vi "Test_Benchmarking_ManyLogEventCall_AvgCallTimeSub50uS.vi"(8 "error in (no error)":errorcluster, 11 "Benchmarking in":refnum<class "Benchmarking.lvclass">) -> (0 "error out":errorcluster, 3 "Benchmarking out":refnum<class "Benchmarking.lvclass">)   [LabVIEW 2017, in "Benchmarking.lvclass"]
uses:
  Benchmarking.lvclass
  Source/Composed Log/LoggerReference/LoggerReference.lvclass/LoggerReference.ctl
  Source/LVQueue Sink/LVQueue Sink.lvclass/LVQueue Sink.ctl
  9d967267-f109-4650-a18c-21849a313d7c.vi
  <vilib>/Analysis/baseanly.llb/Mean (DBL).vi
  9d967267-f109-4650-a18c-21849a313d7c.vi/e70087ac-6783-423e-bbb6-1b0614bba6df.vi
  Source/Composed Log/LoggerReference/Return Aggregate Queues.vi
  Source/Composed Log/LoggerReference/Add Aggregate Log.vi
  9d967267-f109-4650-a18c-21849a313d7c.vi/e70087ac-6783-423e-bbb6-1b0614bba6df.vi/88739b95-52e7-4b20-b235-d6020947c847.vi
  Source/Composed Log/LoggerReference/Send Add Sink.vi
  Source/LVQueue Sink/LVQueue Sink.lvclass
  C:/CS/Internal/LabVIEW/Logger/Source/Composed Log/Log Sink/Log Sink.lvclass
  Source/Composed Log/Application Logger/Launch Worker Loop.vi
  Source/Composed Log/LoggerReference/Initialize Logger Instance.vi
  Source/Composed Log/Singleton Event Log/Logger Queue FGV.vi
  Source/Composed Log/IErrorFormat/IErrorFormat.lvclass
  Source/Composed Log/LoggerReference/LoggerReference.lvclass
  Source/Composed Log/Log Sink/Log Sink.lvclass
  Source/Composed Log/Singleton Event Log/Singleton Event Log.lvlib
  <vilib>/Analysis/NI_AALBase.lvlib
  <vilib>/addons/_JKI Toolkits/VI Tester/TestCase.llb/TestCase.lvclass
  C:/Program Files (x86)/National Instruments/LabVIEW 2017/vi.lib/addons/_JKI Toolkits/VI Tester/TestCase.llb/TestCase.lvclass
panel:
  out "resulting string":string
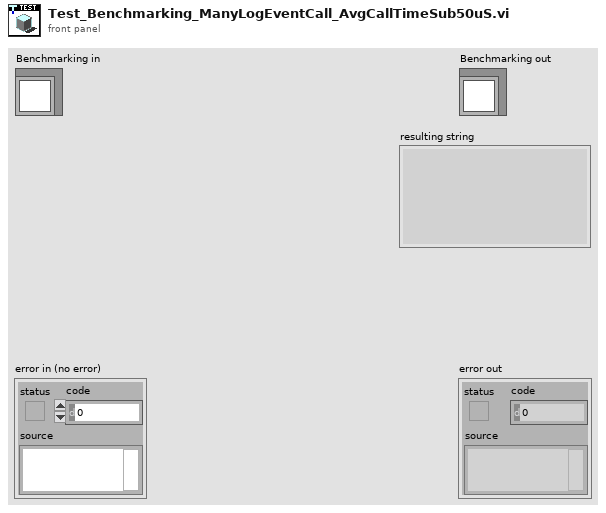
[diagram p1: front panel]
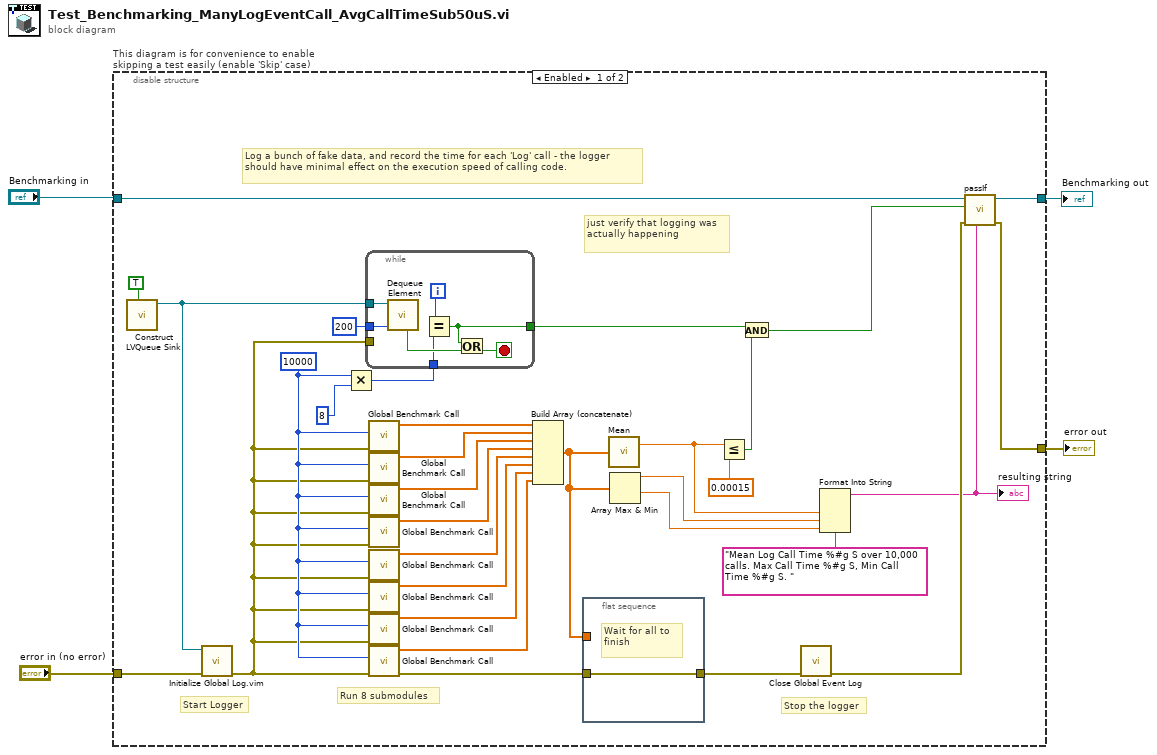
[diagram p0: block diagram]
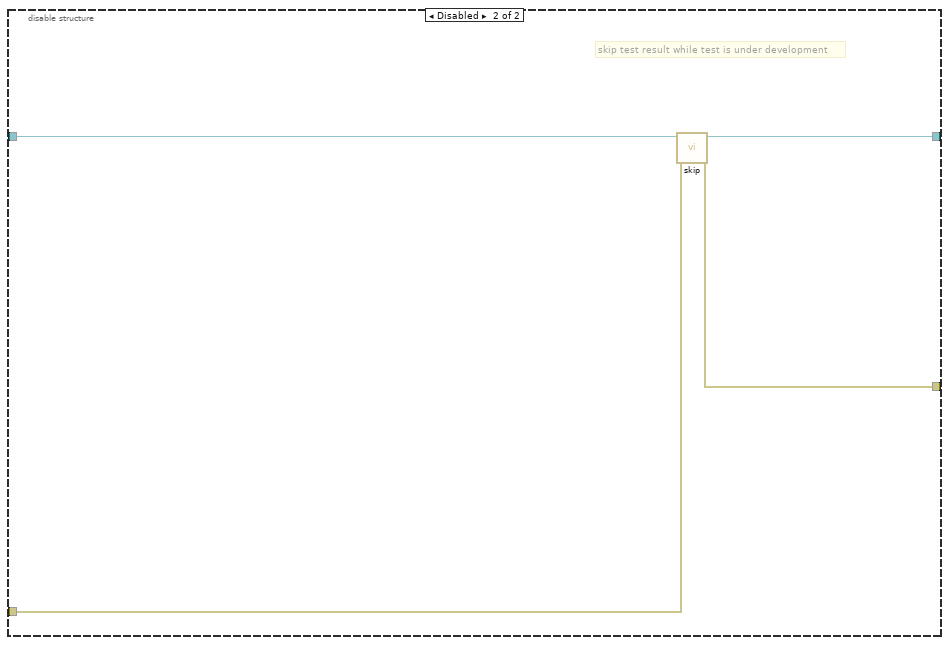
[diagram p2: hidden frame]
diagram:
  n1 = disable-structure "This diagram is for convenience to enable skipping a test easily (enable 'Skip' case)" shown="Enabled" {
    disable-tunnel: "Benchmarking in" -> [w33 w48]
    disable-tunnel: [w32 w46] -> w4
    disable-tunnel: [w34 w47] -> w3
    disable-tunnel: "error in (no error)" -> [w36 w45]
    frame Enabled {
      w14 = 10000 ("Count")
      # "just verify that logging was actually happening"
      # "Run 8 submodules"
      # "Stop the logger"
      # "Start Logger"
      # "Log a bunch of fake data, and record the time for each 'Log' call - the logger should have minimal effect on the execution speed of calling code."
      n2 = call "Construct LVQueue Sink.vi"("User Shutdown? (F)"=TRUE) -> ("LVQueue Sink out"=w16:refnum<class "LVQueue Sink.lvclass">)  [unwired: 9 in, 1 out]
      n3 = call "Initialize Global Log.vim"("error in (no error)"=w36, "Log Sink(s)"=w16) -> ("error out"=w5:errorcluster)  [unwired: 8 in, 1 out]
      n4 = Multiply(x=w14, y=8 ("x")) -> (x*y=w11:i32)
      n5 = while {
        tunnel: w16 -> [w44]
        tunnel: w11 -> [w42]
        tunnel: [w38] -> w10
        tunnel: 200 ("timeout in ms (-1)") -> [w39]
        tunnel: w5 -> [_]
        i -> [w41]
        stop <- w40 stop-if-true
        n6 = call "Dequeue Element.vi"("timeout in ms (-1)"=w39, "LVQueue Sink in"=w44) -> ("Timed Out?"=w43:bool)  [unwired: 6 in, 3 out]
        n7 = Equal?(x=w41, y=w42) -> (x = y?=w38:bool)
        n8 = Or(x=w38, y=w43) -> (x .or. y?=w40:bool)
      }
      n9 = call "Global Benchmark Call.vi"("error in"=w5, "Count"=w14) -> ("Call Times"=w24:dbl[])  [unwired: 8 in, 1 out]
      n10 = call "Global Benchmark Call.vi"("error in"=w5, "Count"=w14) -> ("Call Times"=w23:dbl[])  [unwired: 8 in, 1 out]
      n11 = call "Global Benchmark Call.vi"("error in"=w5, "Count"=w14) -> ("Call Times"=w22:dbl[])  [unwired: 8 in, 1 out]
      n12 = call "Global Benchmark Call.vi"("error in"=w5, "Count"=w14) -> ("Call Times"=w21:dbl[])  [unwired: 8 in, 1 out]
      n13 = call "Global Benchmark Call.vi"("error in"=w5, "Count"=w14) -> ("Call Times"=w20:dbl[])  [unwired: 8 in, 1 out]
      n14 = call "Global Benchmark Call.vi"("error in"=w5, "Count"=w14) -> ("Call Times"=w19:dbl[])  [unwired: 8 in, 1 out]
      n15 = call "Global Benchmark Call.vi"("error in"=w5, "Count"=w14) -> ("Call Times"=w18:dbl[])  [unwired: 8 in, 1 out]
      n16 = call "Global Benchmark Call.vi"("error in"=w5, "Count"=w14) -> ("error out"=w7:errorcluster, "Call Times"=w17:dbl[])  [unwired: 8 in]
      n17 = Build Array (concatenate)(w24, w23, w22, w21, w20, w19, w18, w17) -> (w8:dbl[])
      n18 = flat-sequence {
        tunnel: w8 -> [_]
        tunnel: w7 -> [w37]
        tunnel: [w37] -> w6
        frame #0 {
          # "Wait for all to finish"
        }
      }
      n19 = call-poly <vilib>:"Mean.vi"("X"=w8) -> ("mean"=w28:dbl)  [unwired: 1 out]
      n20 = Array Max & Min(array=w8) -> (max value=w27:dbl, min value=w26:dbl)  [unwired: 2 out]
      n21 = Less Or Equal?(x=w28, y=0.00015) -> (x <= y?=w30:bool)
      n22 = And(x=w10, y=w30) -> (x .and. y?=w12:bool)
      n23 = call "Close Global Event Log.vi"("error in (no error)"=w6) -> ("error out"=w35:errorcluster)  [unwired: 10 in]
      n24 = Format Into String(format string="Mean Log Call Time %#g S over 10,000 calls. Max Call Time %#g S, Min Call Time %#g S. ", w28, w27, w26) -> (resulting string=w25:string)  [unwired: 2 in, 1 out]
      "resulting string" <- w25
      n25 = call-dynamic "passIf.vi"("custom report message (\"\")"=w25, "error in (no error)"=w35, "pass"=w12, "TestCase in"=w33) -> ("error out"=w34:errorcluster, "TestCase out"=w32:refnum<class "Benchmarking.lvclass">)  [unwired: 6 in]
    }
    frame Disabled {
      # "skip test result while test is under development"
      n26 = call <vilib>:"skip.vi"("error in (no error)"=w45, "TestCase in"=w48) -> ("error out"=w47:errorcluster, "TestCase out"=w46:refnum<class "Benchmarking.lvclass">)  [unwired: 8 in]
    }
  }
  "error out" <- w3
  "Benchmarking out" <- w4
